vi "4_5_a.vi"() -> ()   [LabVIEW 2020]
uses:
  <vilib>/numeric/Random Number (Range) U64.vi
  <vilib>/numeric/sub_Random U32.vi
panel:
  out "x-y":u32
  out "Array":u64[](array[numeric])
  in  "Numeric":i32
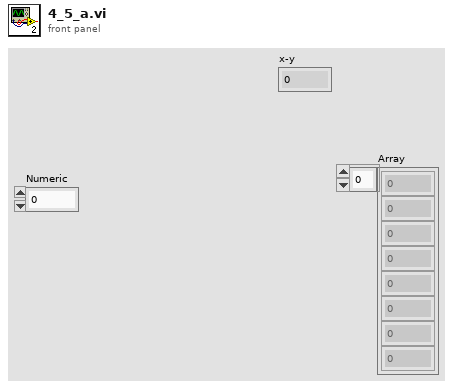
[diagram p1: front panel]
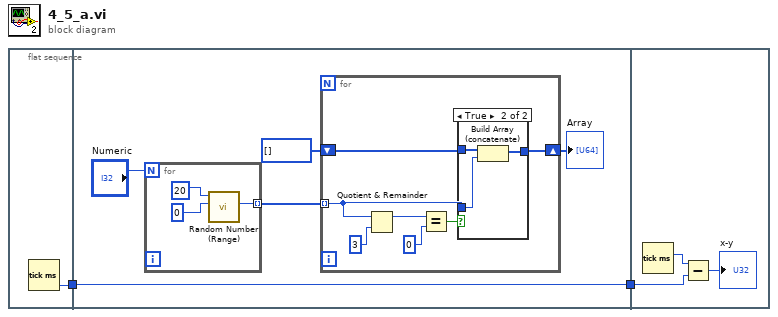
[diagram p0: block diagram]
diagram:
  n1 = flat-sequence {
    tunnel: [w3] -> w2
    tunnel: w2 -> [w4]
    tunnel: [w4] -> w1
    tunnel: w1 -> [w24]
    frame #0 {
      n2 = Tick Count (ms)() -> (millisecond timer value=w3:u32)
    }
    frame #1 {
      n3 = for {
        N: "Numeric" -> [_]
        tunnel: [w20] -> w7 mode=indexing
        n4 = call-poly <vilib>:"Random Number (Range).vi"("lower bound (0)"=u64 0, "upper bound (100)"=u64 20) -> ("number"=w20:u64)  [unwired: 9 in]
      }
      n5 = for {
        tunnel: w7 -> [w9] mode=indexing
        shift-right: [w11] -> w6
        shift-left: u64[] [] -> [w10]
        n6 = Quotient & Remainder(x=w9, y=u64 3) -> (x-y*floor(x/y)=w14:u64)  [unwired: 1 out]
        n7 = Equal?(x=w14, y=u64 0) -> (x = y?=w12:bool)
        n8 = case shown="True" w12 {
          tunnel: w9 -> [_ w19]
          tunnel: [w16 w18] -> w11
          tunnel: w10 -> [w16 w17]
          frame False {
          }
          frame True {
            n9 = Build Array (concatenate)(w17, w19) -> (w18:u64[])
          }
        }
      }
      "Array" <- w6
    }
    frame #2 {
      n10 = Tick Count (ms)() -> (millisecond timer value=w25:u32)
      n11 = Subtract(x=w25, y=w24) -> (x-y=→"x-y":u32)
    }
  }
